vi "spring.vi"(7 "action (set itemstrings)":T2=enum."set itemstrings", 8 "error in (no error)":errorcluster, 9 "indentation/item symbols/colors in":u32[](array[numeric]), 10 "item strings in":string[][](array[string]), 11 "tree ref":refnum<vi>) -> (0 "error out":errorcluster, 1 "item symbols/colors out":u32[](array[numeric]), 2 "item strings out":string[][](array[string]))   [LabVIEW 2015]
uses:
  spring action.ctl
  spring - node data.ctl
panel:
  out "Cluster":cluster{"bolded?":bool}
  in  "node data":cluster{T1[]}
  # "If you get error 16,\nthe number of columns\nin the input and tree\ndoes not match."
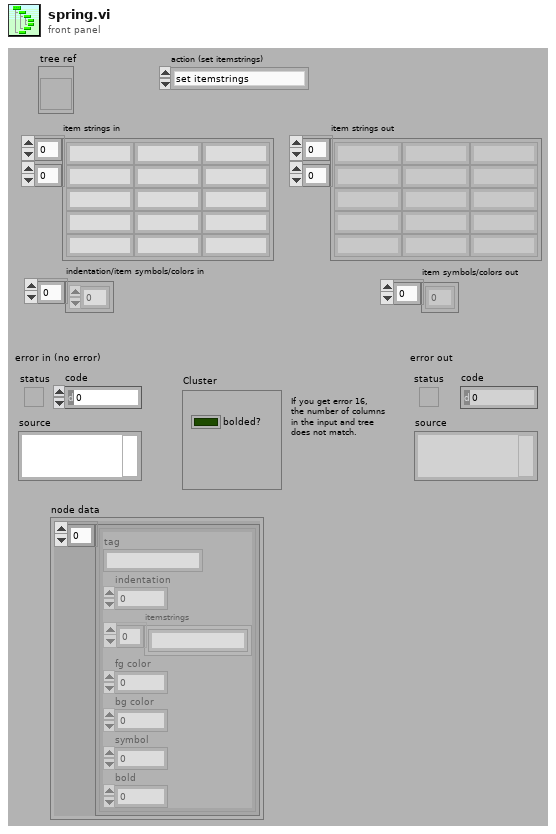
[diagram p1: front panel]
types:
  T1 = typedef "spring - node data.ctl" = cluster{"tag":string, "indentation":i32, "itemstrings":string[], "fg color":u32, "bg color":u32, "symbol":u32, "bold":u32}
  T2 = typedef "spring action.ctl" = enum16{"_init", "_add tree", "set itemstrings", "set fg colors", "set bg colors", "set symbols", "get tags", "get itemstrings", "get fg colors", "get bg colors", "get symbols", "empty tree", "update from tree", "find index of tag(s)", "set bold"}
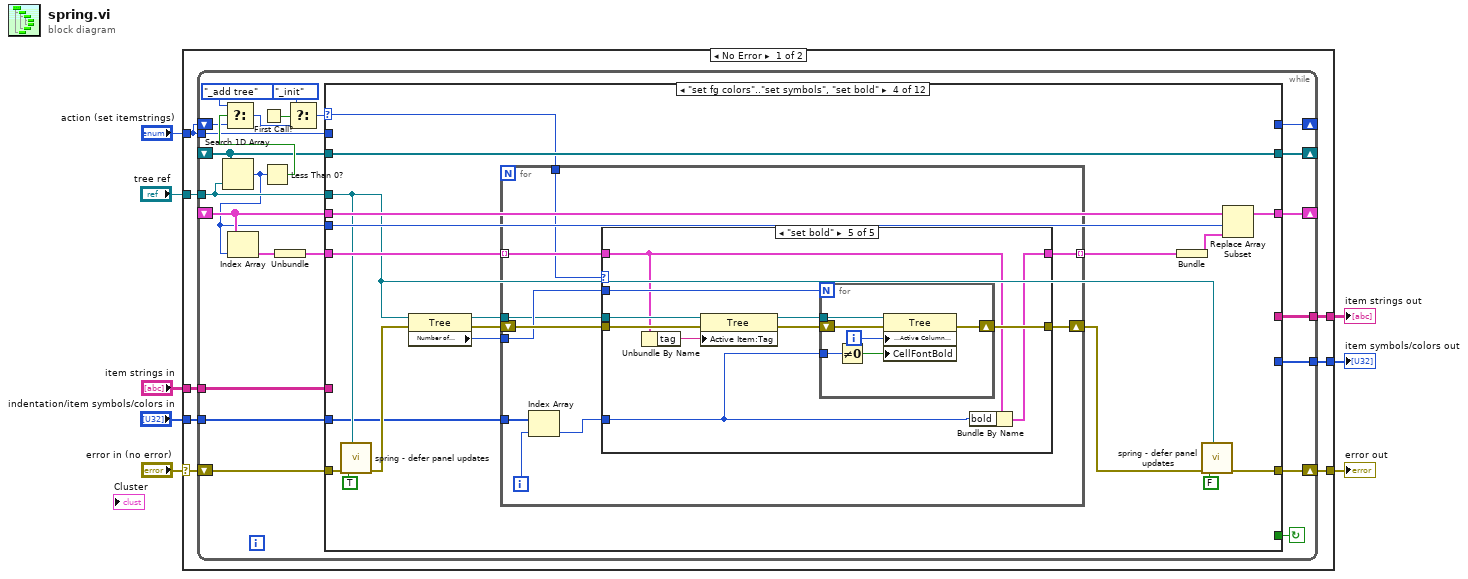
[diagram p0: block diagram]
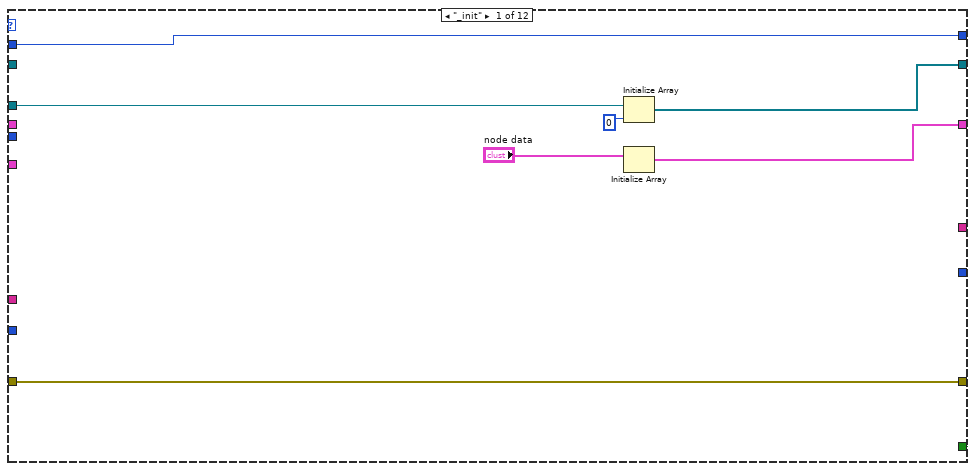
[diagram p2: hidden frame]
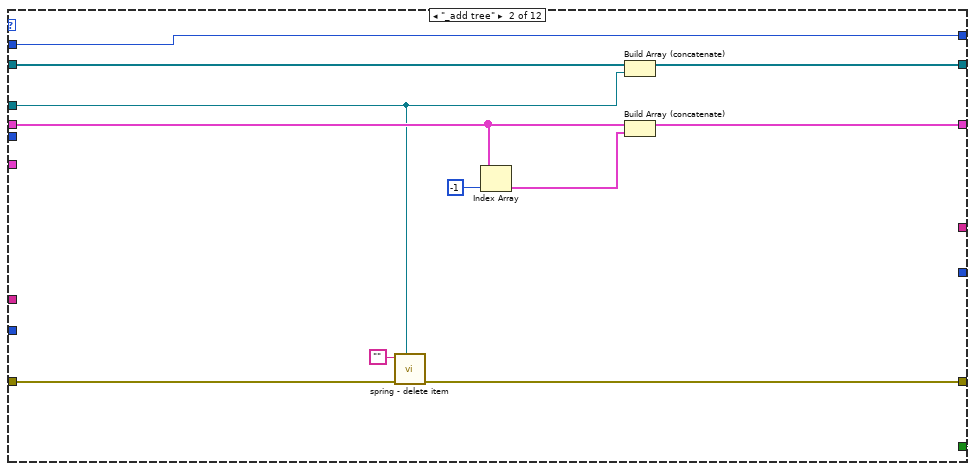
[diagram p3: hidden frame]
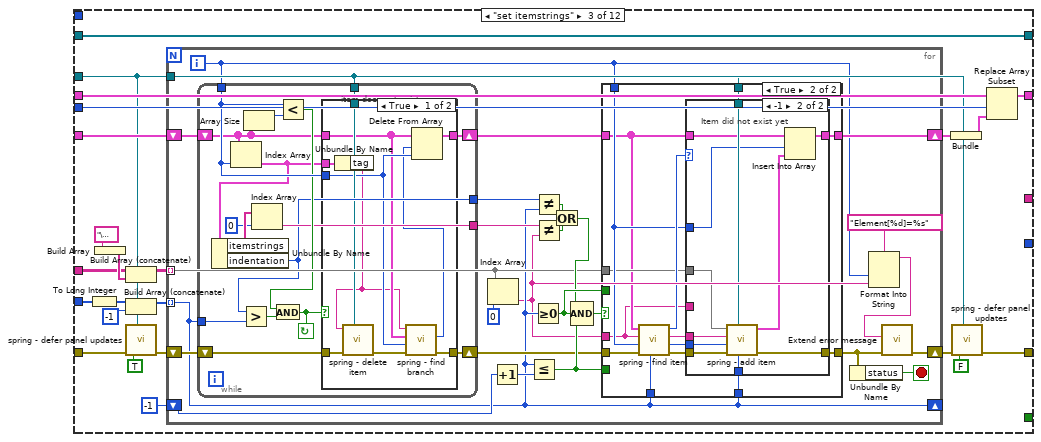
[diagram p4: hidden frame]
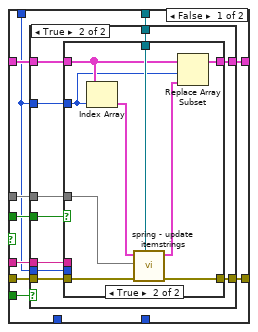
[diagram p6: hidden frame]
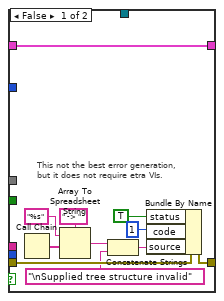
[diagram p7: hidden frame]
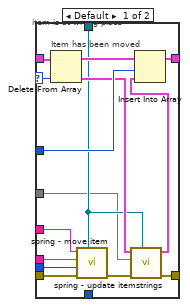
[diagram p9: hidden frame]
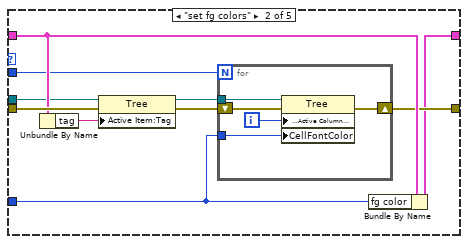
[diagram p11: hidden frame]
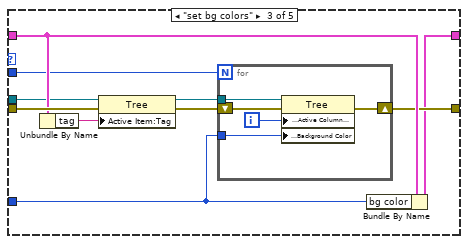
[diagram p12: hidden frame]
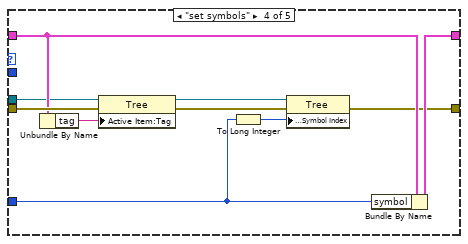
[diagram p13: hidden frame]
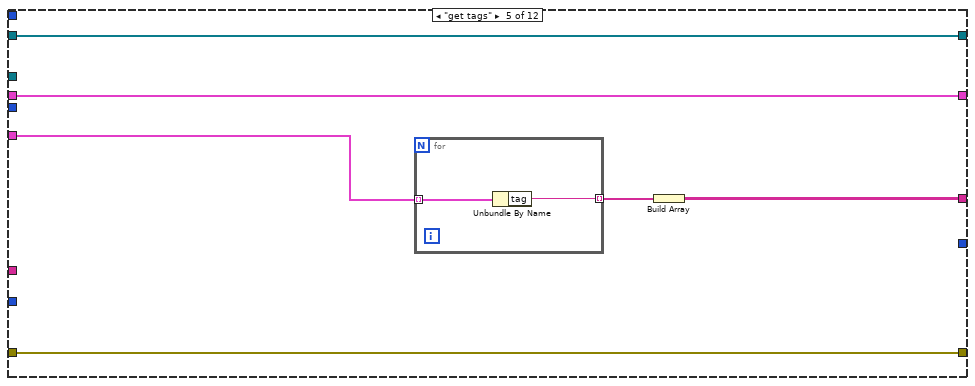
[diagram p14: hidden frame]
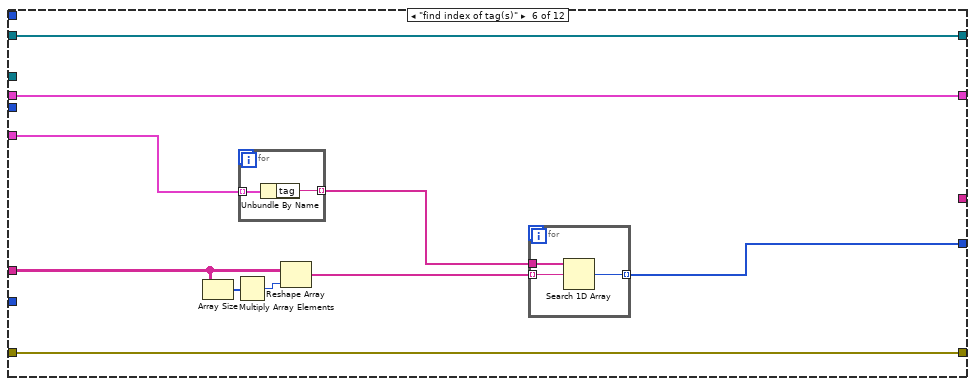
[diagram p15: hidden frame]
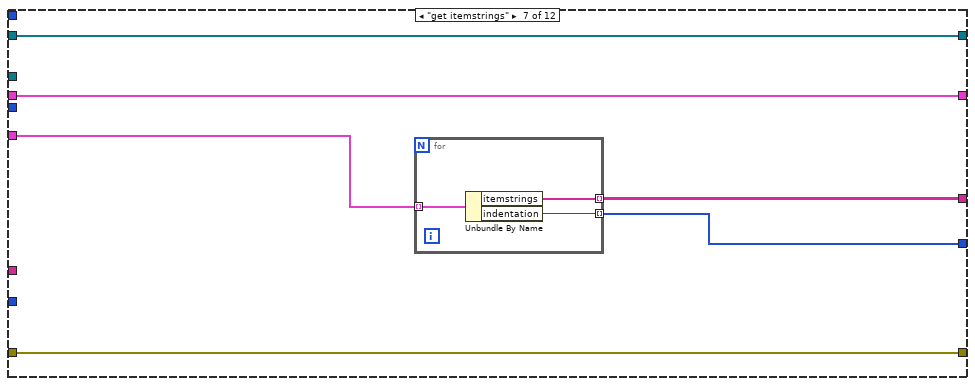
[diagram p16: hidden frame]
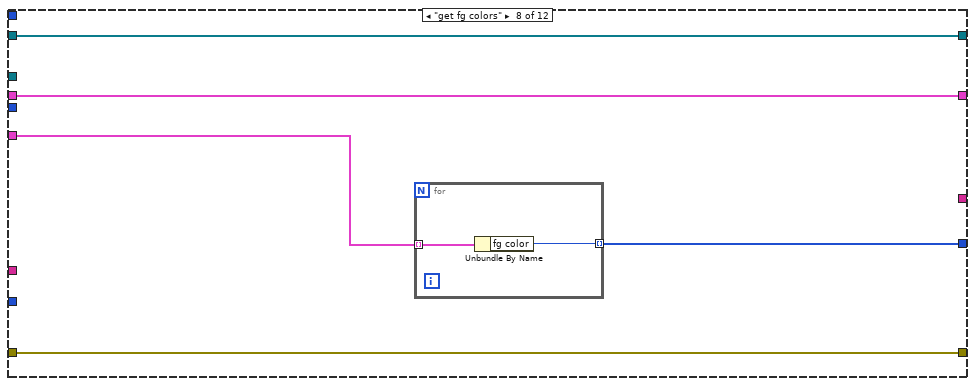
[diagram p17: hidden frame]
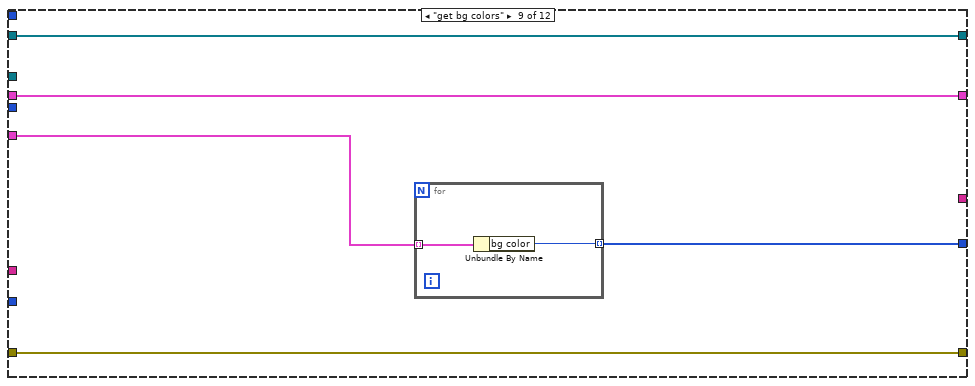
[diagram p18: hidden frame]
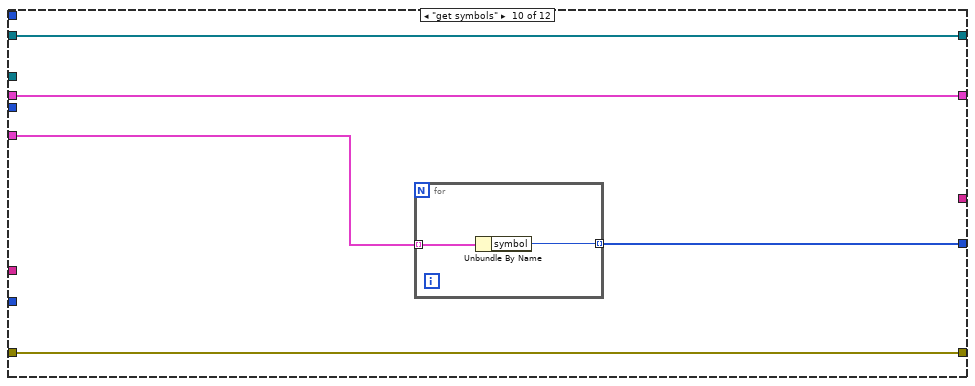
[diagram p19: hidden frame]
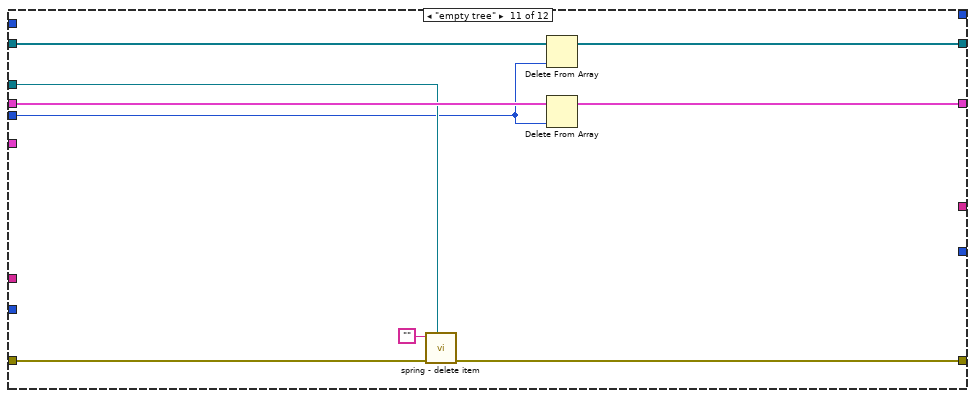
[diagram p20: hidden frame]
diagram:
  n1 = case shown="No Error" "error in (no error)" {
    selector: "error in (no error)" -> [w15 w410]
    tunnel: "tree ref" -> [w16 _]
    tunnel: [w14 w410] -> w6
    tunnel: "item strings in" -> [w13 _]
    tunnel: "action (set itemstrings)" -> [w12 _]
    tunnel: [w11 _] -> w3
    tunnel: "indentation/item symbols/colors in" -> [w10 _]
    tunnel: [w9 _] -> w1
    frame No Error {
      n2 = while {
        tunnel: w16 -> [w30]
        shift-right: [w29] -> _
        shift-left: _ -> [w28]
        shift-right: [w39] -> w14
        shift-left: w15 -> [w40]
        tunnel: w13 -> [w27]
        shift-right: [w32] -> _
        shift-left: w12 -> [w33]
        tunnel: w12 -> [w31]
        shift-right: [w25] -> _
        shift-left: _ -> [w24]
        tunnel: [w21] -> w11
        tunnel: w10 -> [w18]
        tunnel: [w17] -> w9
        stop <- w26 continue-if-true
        n3 = Search 1D Array(1D array=w28, element=w30) -> (index of element=w22:i32)  [unwired: 1 in]
        n4 = Index Array(array=w24, index=w22) -> (element=w20:cluster{T1[]})
        n5 = First Call?() -> (First Call?: T/F=w37:bool)
        n6 = Less Than 0?(x=w22) -> (x < 0?=w36:bool)
        n7 = Select(t=spring_action."_add tree" ("action"), s=w36, f=w33) -> (s? t:f=w38:T2)
        n8 = Unbundle(w20) -> (w19:T1[])
        n9 = Select(t=spring_action."_init" ("action"), s=w37, f=w38) -> (s? t:f=w35:T2)
        n10 = case shown="\"set fg colors\"..\"set symbols\", \"set bold\"" w35 {
          selector: w35 -> [_ _ _ w227 _ _ _ _ _ _ _ _]
          tunnel: w40 -> [w43 w51 w62 w233 w310 w322 w333 w341 w348 w355 w365 w382]
          tunnel: [w43 w49 w68 w220 w310 w322 w333 w341 w348 w355 w364 w371] -> w39
          tunnel: [w48 w57 _ _ _ _ _ _ _ _ _ _] -> w32
          tunnel: w31 -> [w48 w57 _ _ _ _ _ _ _ _ _ _]
          tunnel: w30 -> [w46 w52 w64 w225 _ _ _ _ _ _ w366 w380]
          tunnel: [w47 w60 w83 w238 w311 w323 w334 w342 w349 w356 w360 w387] -> w29
          tunnel: w28 -> [_ w59 w83 w238 w311 w323 w334 w342 w349 w356 w361 w387]
          tunnel: w27 -> [_ _ w63 _ _ w315 _ _ _ _ _ _]
          tunnel: [TRUE TRUE _ _ _ _ _ _ _ _ _ _] -> w26
          tunnel: w22 -> [_ _ w80 w235 _ _ _ _ _ _ w362 w384]
          tunnel: w24 -> [_ w54 w81 w236 w312 w324 w335 w343 w350 w357 w368 w385]
          tunnel: [w41 w58 w82 w237 w312 w324 w335 w343 w350 w357 w367 w386] -> w25
          tunnel: [_ _ _ _ w308 _ w331 _ _ _ _ w370] -> w21
          tunnel: w19 -> [_ _ w72 w231 w309 w321 w332 w340 w347 w354 _ w374]
          tunnel: w18 -> [_ _ w67 w223 _ _ _ _ _ _ _ _]
          tunnel: [_ _ _ _ _ w319 w330 w339 w346 w353 _ w369] -> w17
          frame "_init" {
            n11 = Initialize Array(w46, 0 ("dimension size")) -> (w47:refnum<vi>[])
            n12 = Initialize Array("node data") -> (w41:cluster{T1[]}[])  [unwired: 1 in]
          }
          frame "_add tree" {
            n13 = call "spring - delete item.vi"("tree ref"=w52, "error in (no error)"=w51, "tag"="") -> ("error out"=w49:errorcluster)  [unwired: 8 in]
            n14 = Index Array(array=w54, index=-1) -> (element=w53:cluster{T1[]})
            n15 = Build Array (concatenate)(w59, w52) -> (w60:refnum<vi>[])
            n16 = Build Array (concatenate)(w54, w53) -> (w58:cluster{T1[]}[])
          }
          frame "set itemstrings" {
            n17 = To Long Integer(number=w67) -> (32bit integer=w61:i32[])
            n18 = Build Array("\u0000" ("String")) -> (w77:string[])
            n19 = Build Array (concatenate)(w63, w77) -> (w78:string[][])
            n20 = Build Array (concatenate)(w61, -1 ("disabled index (col)")) -> (w66:i32[])
            n21 = call "spring - defer panel updates.vi"("tree ref"=w64, "error in (no error) (will be ignored)"=w62, "defer panel updates"=TRUE ("enable panel updates")) -> ("error out"=w75:errorcluster)  [unwired: 8 in]
            n22 = for {
              shift-right: [w88] -> w69
              shift-left: w75 -> [w99]
              tunnel: w64 -> [w104]
              tunnel: w78 -> [w93] mode=indexing
              shift-right: [w109] -> w71
              shift-left: w72 -> [w108]
              shift-right: [w92] -> _
              shift-left: -1 ("indentation") -> [w103]
              tunnel: w66 -> [w92] mode=indexing
              i -> [w87]
              stop <- w89 stop-if-true
              n23 = while {
                tunnel: w104 -> [w123]
                shift-right: [w125] -> w107
                shift-left: w108 -> [w115]
                shift-right: [w124] -> w98
                shift-left: w99 -> [w122]
                tunnel: w87 -> [w118]
                tunnel: [w111] -> w106
                tunnel: w92 -> [w120]
                tunnel: [w110] -> w94
                stop <- w119 continue-if-true
                n24 = Index Array(array=w115, index=w118) -> (element=w114:T1)
                n25 = Unbundle By Name(w114) -> ("itemstrings"=w113:string[], "indentation"=w110:i32)
                n26 = Greater?(x=w110, y=w120) -> (0:w121:bool)
                n27 = Array Size(array=w115) -> (size(s)=w117:i32)
                n28 = Index Array(array=w113, index=0) -> (element=w111:string)
                n29 = Less?(x=w118, y=w117) -> (x < y?=w116:bool)
                n30 = And(x=w116, y=w121) -> (x .and. y?=w119:bool)
                n31 = case shown="True" w119 {
                  tunnel: w115 -> [w128 w137]
                  tunnel: w122 -> [w135 w136]
                  tunnel: [w133 w136] -> w124
                  tunnel: w123 -> [w132 _]
                  tunnel: [w131 w137] -> w125
                  tunnel: w118 -> [w130 _]
                  tunnel: w114 -> [w129 _]
                  frame True {
                    # "item does not exist anymore"
                    n32 = Unbundle By Name(w129) -> ("tag"=w127:string)
                    n33 = call "spring - delete item.vi"("tree ref"=w132, "error in (no error)"=w135, "tag"=w127) -> ("error out"=w134:errorcluster)  [unwired: 8 in]
                    n34 = call "spring - find branch.vi"("error in (no error)"=w134, "branch index"=w130, "tree data"=w128, "tag"=w127) -> ("error out"=w133:errorcluster, "branch size"=w126:i32)  [unwired: 6 in]
                    n35 = Delete From Array(array=w128, length=w126, index=w130) -> (array with subset deleted=w131:T1[])  [unwired: 1 out]
                  }
                  frame False {
                  }
                }
              }
              n36 = Index Array(array=w93, index=0) -> (element=w84:string)
              n37 = Increment(x=w103) -> (x+1=w102:i32)
              n38 = Less Or Equal?(x=w92, y=w102) -> (x <= y?=w101:bool)
              n39 = Greater Or Equal To 0?(x=w92) -> (x >= 0?=w100:bool)
              n40 = Not Equal?(x=w94, y=w92) -> (x != y?=w95:bool)
              n41 = Not Equal?(x=w106, y=w84) -> (x != y?=w97:bool)
              n42 = Or(x=w95, y=w97) -> (x .or. y?=w96:bool)
              n43 = Compound Arithmetic op=AND(w96, w100, w101) -> (w105:bool)
              n44 = case shown="True" w105 {
                tunnel: w107 -> [w144 w186]
                tunnel: w98 -> [w146 w190]
                tunnel: [w145 w193] -> w90
                tunnel: w104 -> [w141 w192]
                tunnel: [w143 w191] -> w109
                tunnel: w87 -> [w138 w188]
                tunnel: w93 -> [w140 w187]
                tunnel: w101 -> [w147 _]
                tunnel: w84 -> [w142 w185]
                tunnel: w100 -> [w139 _]
                tunnel: w92 -> [_ w184]
                tunnel: w92 -> [_ w180]
                frame False {
                  n45 = case shown="True" w147 {
                    tunnel: w146 -> [w158 w168]
                    tunnel: [w157 w164] -> w145
                    tunnel: w144 -> [w148 w167]
                    tunnel: [w148 w162] -> w143
                    tunnel: w142 -> [_ w166]
                    tunnel: w138 -> [_ w165]
                    tunnel: w141 -> [_ w163]
                    tunnel: w140 -> [_ w161]
                    tunnel: w139 -> [_ w160]
                    tunnel: w138 -> [_ w159]
                    frame False {
                      # "This not the best error generation,\nbut it does not require etra VIs."
                      n46 = Call Chain() -> (call chain=w154:string[])
                      n47 = Array To Spreadsheet String(delimiter (Tab)=" -> ", array=w154, 3:"%s" ("format string")) -> (spreadsheet string=w150:string)
                      n48 = Concatenate Strings(w150, "\nSupplied tree structure invalid" ("format string")) -> (w151:string)
                      n49 = Bundle By Name(cluster=w158, "status"=TRUE, "code"=1, "source"=w151) -> (w157:errorcluster)
                    }
                    frame True {
                      n50 = case shown="True" w160 {
                        tunnel: w168 -> [w169 w174]
                        tunnel: w167 -> [w170 w173]
                        tunnel: w166 -> [_ _]
                        tunnel: w165 -> [_ _]
                        tunnel: [w169 w179] -> w164
                        tunnel: w163 -> [_ w177]
                        tunnel: [w170 w176] -> w162
                        tunnel: w161 -> [_ w175]
                        tunnel: w159 -> [_ w171]
                        frame False {
                          # "We've encountered the dummy \\00 item that was prepended at the start."
                        }
                        frame True {
                          n51 = Index Array(array=w173, index=w171) -> (element=w172:T1)
                          n52 = call "spring - update itemstrings.vi"("tree ref"=w177, "error in (no error)"=w174, "itemstrings"=w175, "node data"=w172) -> ("error out"=w179:errorcluster, "node data out"=w178:T1)  [unwired: 6 in]
                          n53 = Replace Array Subset(array=w173, new element=w178, index=w171) -> (w176:T1[])
                        }
                      }
                    }
                  }
                }
                frame True {
                  n54 = call "spring - find item.vi"("indentation"=w184, "error in (no error)"=w190, "item index"=w188, "primary itemstring to be found"=w185, "tree data"=w186) -> ("error out"=w181:errorcluster, "son# (0=first)"=w183:i32, "parent tag"=w182:string, "moved item's index"=w189:i32)  [unwired: 3 in]
                  n55 = case shown="-1" w189 {
                    selector: w189 -> [w204 _]
                    tunnel: w186 -> [w207 w216]
                    tunnel: w181 -> [w208 w214]
                    tunnel: [w201 w219] -> w193
                    tunnel: w192 -> [w197 w218]
                    tunnel: [w205 w217] -> w191
                    tunnel: w188 -> [w203 w215]
                    tunnel: w187 -> [w196 w209]
                    tunnel: w185 -> [w198 _]
                    tunnel: w183 -> [w195 w212]
                    tunnel: w182 -> [w194 w210]
                    tunnel: w180 -> [_ w211]
                    frame Default {
                      # "Item has been moved"
                      # "item is at wrong place"
                      n56 = Delete From Array(array=w207, index=w204) -> (deleted portion=w200:T1, array with subset deleted=w206:T1[])  [unwired: 1 in]
                      n57 = call "spring - move item.vi"("tree ref"=w197, "error in (no error)"=w208, "position (0=just below parent etc.)"=w195, "parent tag"=w194, "tag"=w198) -> ("error out"=w202:errorcluster)  [unwired: 6 in]
                      n58 = call "spring - update itemstrings.vi"("tree ref"=w197, "error in (no error)"=w202, "itemstrings"=w196, "node data"=w200) -> ("error out"=w201:errorcluster, "node data out"=w199:T1)  [unwired: 6 in]
                      n59 = Insert Into Array(array=w206, index=w203, new element=w199) -> (w205:T1[])
                    }
                    frame -1 {
                      # "Item did not exist yet"
                      n60 = call "spring - add item.vi"("new indentation"=w211, "tree ref"=w218, "error in (no error)"=w214, "position (0=just below parent etc.)"=w212, "parent tag"=w210, "itemstrings"=w209) -> ("error out"=w219:errorcluster, "node data out"=w213:T1)  [unwired: 4 in]
                      n61 = Insert Into Array(array=w216, index=w215, new element=w213) -> (w217:T1[])
                    }
                  }
                }
              }
              n62 = Unbundle By Name(w90) -> ("status"=w89:bool)
              n63 = Format Into String(format string="Element[%d]=%s", w87, w84) -> (resulting string=w85:string)  [unwired: 2 in, 1 out]
              n64 = call "Extend error message.vi"("error in"=w90, "extra message part"=w85) -> ("error out"=w88:errorcluster)  [unwired: 9 in]
            }
            n65 = Bundle(w71) -> (w79:cluster{T1[]})  [unwired: 1 in]
            n66 = call "spring - defer panel updates.vi"("tree ref"=w64, "error in (no error) (will be ignored)"=w69, "defer panel updates"=FALSE ("enable panel updates")) -> ("error out"=w68:errorcluster)  [unwired: 8 in]
            n67 = Replace Array Subset(array=w81, new element=w79, index=w80) -> (w82:cluster{T1[]}[])
          }
          frame "set fg colors".."set symbols", "set bold" {
            n68 = call "spring - defer panel updates.vi"("tree ref"=w225, "error in (no error) (will be ignored)"=w233, "defer panel updates"=TRUE ("enable panel updates")) -> ("error out"=w228:errorcluster)  [unwired: 8 in]
            n69 = property on="Property Node" class="Tree"(reference=w225, error in=w228) -> (reference out=w224:refnum<vi>, error out=w229:errorcluster, "Number of Columns"=w230:u32)
            n70 = for {
              shift-right: [w245] -> w221
              shift-left: w229 -> [w248]
              tunnel: w224 -> [w242]
              tunnel: w231 -> [w247] mode=indexing
              tunnel: w230 -> [w246]
              tunnel: w227 -> [w243]
              tunnel: [w244] -> w226 mode=indexing
              tunnel: w223 -> [w241]
              i -> [w240]
              n71 = Index Array(array=w241, index=w240) -> (element=w239:u32)
              n72 = case shown="\"set bold\"" w243 {
                tunnel: w248 -> [w250 w260 w275 w290 w296]
                tunnel: w247 -> [w249 w258 w273 w289 w293]
                tunnel: w246 -> [_ w251 w272 _ w295]
                tunnel: [w250 w257 w271 w283 w294] -> w245
                tunnel: [w249 w256 w270 w288 w291] -> w244
                tunnel: w239 -> [_ w254 w268 w282 w292]
                tunnel: w242 -> [_ w252 w266 w286 w297]
                frame Default {
                  # "should never be reached"
                }
                frame "set fg colors" {
                  n73 = Unbundle By Name(w258) -> ("tag"=w255:string)
                  n74 = property on="Property Node" class="Tree"(reference=w252, error in=w260, "Active Item:Tag"=w255) -> (reference out=w253:refnum<vi>, error out=w259:errorcluster)
                  n75 = for {
                    N: w251 -> [_]
                    shift-right: [w263] -> w257
                    shift-left: w259 -> [w265]
                    tunnel: w254 -> [w262]
                    tunnel: w253 -> [w261]
                    i -> [w264]
                    n76 = property on="Property Node" class="Tree"(reference=w261, error in=w265, "Active Cell:Active Column Number"=w264, "CellFontColor"=w262) -> (error out=w263:errorcluster)  [unwired: 1 out]
                  }
                  n77 = Bundle By Name(cluster=w258, "fg color"=w254) -> (w256:T1)
                }
                frame "set bg colors" {
                  n78 = Unbundle By Name(w273) -> ("tag"=w269:string)
                  n79 = property on="Property Node" class="Tree"(reference=w266, error in=w275, "Active Item:Tag"=w269) -> (reference out=w267:refnum<vi>, error out=w274:errorcluster)
                  n80 = for {
                    N: w272 -> [_]
                    shift-right: [w278] -> w271
                    shift-left: w274 -> [w280]
                    tunnel: w268 -> [w277]
                    tunnel: w267 -> [w276]
                    i -> [w279]
                    n81 = property on="Property Node" class="Tree"(reference=w276, error in=w280, "Active Cell:Active Column Number"=w279, "Active Cell:Background Color"=w277) -> (error out=w278:errorcluster)  [unwired: 1 out]
                  }
                  n82 = Bundle By Name(cluster=w273, "bg color"=w268) -> (w270:T1)
                }
                frame "set symbols" {
                  n83 = Unbundle By Name(w289) -> ("tag"=w287:string)
                  n84 = property on="Property Node" class="Tree"(reference=w286, error in=w290, "Active Item:Tag"=w287) -> (reference out=w285:refnum<vi>, error out=w284:errorcluster)
                  n85 = To Long Integer(number=w282) -> (32bit integer=w281:i32)
                  n86 = property on="Property Node" class="Tree"(reference=w285, error in=w284, "Active Item:Symbol Index"=w281) -> (error out=w283:errorcluster)  [unwired: 1 out]
                  n87 = Bundle By Name(cluster=w289, "symbol"=w282) -> (w288:T1)
                }
                frame "set bold" {
                  n88 = Unbundle By Name(w293) -> ("tag"=w299:string)
                  n89 = property on="Property Node" class="Tree"(reference=w297, error in=w296, "Active Item:Tag"=w299) -> (reference out=w298:refnum<vi>, error out=w300:errorcluster)
                  n90 = for {
                    N: w295 -> [_]
                    shift-right: [w304] -> w294
                    shift-left: w300 -> [w306]
                    tunnel: w298 -> [w303]
                    tunnel: w292 -> [w301]
                    i -> [w305]
                    n91 = Not Equal To 0?(x=w301) -> (x != 0?=w302:bool)
                    n92 = property on="Property Node" class="Tree"(reference=w303, error in=w306, "Active Cell:Active Column Number"=w305, "CellFontBold"=w302) -> (error out=w304:errorcluster)  [unwired: 1 out]
                  }
                  n93 = Bundle By Name(cluster=w293, "bold"=w292) -> (w291:T1)
                }
              }
            }
            n94 = Bundle(w226) -> (w234:cluster{T1[]})  [unwired: 1 in]
            n95 = call "spring - defer panel updates.vi"("tree ref"=w225, "error in (no error) (will be ignored)"=w221, "defer panel updates"=FALSE ("enable panel updates")) -> ("error out"=w220:errorcluster)  [unwired: 8 in]
            n96 = Replace Array Subset(array=w236, new element=w234, index=w235) -> (w237:cluster{T1[]}[])
          }
          frame "get tags" {
            n97 = for {
              tunnel: w309 -> [w314] mode=indexing
              tunnel: [w313] -> w307 mode=indexing
              n98 = Unbundle By Name(w314) -> ("tag"=w313:string)
            }
            n99 = Build Array(w307) -> (w308:string[][])
          }
          frame "find index of tag(s)" {
            n100 = Array Size(array=w315) -> (size(s)=w317:i32[])
            n101 = Multiply Array Elements(1:w317) -> (0:w316:i32)
            n102 = for {
              tunnel: w321 -> [w329] mode=indexing
              tunnel: [w328] -> w320 mode=indexing
              n103 = Unbundle By Name(w329) -> ("tag"=w328:string)
            }
            n104 = Reshape Array(w315, w316) -> (w318:string[])
            n105 = for {
              tunnel: w320 -> [w327]
              tunnel: w318 -> [w326] mode=indexing
              tunnel: [w325] -> w319 mode=indexing
              n106 = Search 1D Array(1D array=w327, element=w326) -> (index of element=w325:i32)  [unwired: 1 in]
            }
          }
          frame "get itemstrings" {
            n107 = for {
              tunnel: w332 -> [w338] mode=indexing
              tunnel: [w337] -> w331 mode=indexing
              tunnel: [w336] -> w330 mode=indexing
              n108 = Unbundle By Name(w338) -> ("itemstrings"=w337:string[], "indentation"=w336:i32)
            }
          }
          frame "get fg colors" {
            n109 = for {
              tunnel: w340 -> [w345] mode=indexing
              tunnel: [w344] -> w339 mode=indexing
              n110 = Unbundle By Name(w345) -> ("fg color"=w344:u32)
            }
          }
          frame "get bg colors" {
            n111 = for {
              tunnel: w347 -> [w352] mode=indexing
              tunnel: [w351] -> w346 mode=indexing
              n112 = Unbundle By Name(w352) -> ("bg color"=w351:u32)
            }
          }
          frame "get symbols" {
            n113 = for {
              tunnel: w354 -> [w359] mode=indexing
              tunnel: [w358] -> w353 mode=indexing
              n114 = Unbundle By Name(w359) -> ("symbol"=w358:u32)
            }
          }
          frame "empty tree" {
            n115 = call "spring - delete item.vi"("tree ref"=w366, "error in (no error)"=w365, "tag"="") -> ("error out"=w364:errorcluster)  [unwired: 8 in]
            n116 = Delete From Array(array=w361, index=w362) -> (array with subset deleted=w360:refnum<vi>[])  [unwired: 1 in, 1 out]
            n117 = Delete From Array(array=w368, index=w362) -> (array with subset deleted=w367:cluster{T1[]}[])  [unwired: 1 in, 1 out]
          }
          frame "update from tree" {
            n118 = call "spring - defer panel updates.vi"("tree ref"=w380, "error in (no error) (will be ignored)"=w382, "defer panel updates"=TRUE ("enable panel updates")) -> ("error out"=w378:errorcluster)  [unwired: 8 in]
            n119 = property on="Property Node" class="Tree"(reference=w380, error in=w378) -> (error out=w377:errorcluster, "Displayed Items"=w379:string[], "Number of Columns"=w376:u32)  [unwired: 1 out]
            n120 = for {
              shift-right: [w400] -> w372
              shift-left: w377 -> [w401]
              tunnel: w380 -> [w399]
              tunnel: w379 -> [w390] mode=indexing
              tunnel: w376 -> [w404]
              tunnel: [w395] -> w375 mode=indexing
              tunnel: w374 -> [w397]
              tunnel: [w389] -> w370 mode=indexing
              tunnel: [w388] -> w369 mode=indexing
              (unwired) 0 ("index")
              n121 = property on="Property Node" class="Tree"(reference=w399, error in=w401, "Active Item:Tag"=w390, "Active Cell:Active Column Number"=0 ("Active Cell Properties:Active Column Number")) -> (reference out=w403:refnum<vi>, error out=w402:errorcluster, "Active Item:Indent Level"=w388:i32, "Active Item:Symbol Index"=w394:i32, "Active Cell:Background Color"=w392:u32, "Active Cell:Foreground Color"=w391:u32)
              n122 = for {
                N: w404 -> [_]
                tunnel: w403 -> [w409]
                tunnel: [w405] -> w389 mode=indexing
                shift-right: [w406] -> w400
                shift-left: w402 -> [w407]
                i -> [w408]
                n123 = property on="Property Node" class="Tree"(reference=w409, error in=w407, "Active Cell:Active Column Number"=w408) -> (error out=w406:errorcluster, "Active Cell:String"=w405:string)  [unwired: 1 out]
              }
              n124 = Index Array(array=w397, index=-1) -> (element=w396:T1)
              n125 = Bundle By Name(cluster=w396, "tag"=w390, "indentation"=w388, "symbol"=w394, "bg color"=w392, "fg color"=w391, "itemstrings"=w389) -> (w395:T1)
            }
            n126 = call "spring - defer panel updates.vi"("tree ref"=w380, "error in (no error) (will be ignored)"=w372, "defer panel updates"=FALSE ("enable panel updates")) -> ("error out"=w371:errorcluster)  [unwired: 8 in]
            n127 = Bundle(w375) -> (w383:cluster{T1[]})  [unwired: 1 in]
            n128 = Replace Array Subset(array=w385, new element=w383, index=w384) -> (w386:cluster{T1[]}[])
          }
        }
      }
    }
    frame Error {
    }
  }
  "error out" <- w6
  "item strings out" <- w3
  "item symbols/colors out" <- w1
